vi "trace_init.vi"() -> (1 "Init seq.":string)   [LabVIEW 2021]
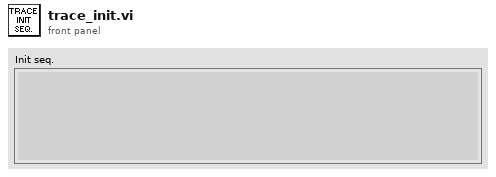
[diagram p1: front panel]
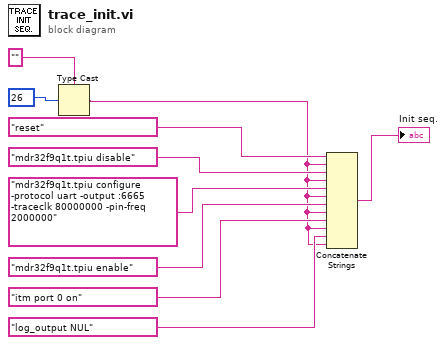
[diagram p0: block diagram]
diagram:
  n1 = Type Cast(type="", x=u8 26) -> (*(type *) &x=w1:string)
  n2 = Concatenate Strings("reset" ("data in"), w1, "mdr32f9q1t.tpiu disable" ("data in"), w1, "mdr32f9q1t.tpiu configure -protocol uart -output :6665 -traceclk 80000000 -pin-freq 2000000" ("data in"), w1, "mdr32f9q1t.tpiu enable" ("data in"), w1, "itm port 0 on" ("data in"), w1, "log_output NUL" ("data in"), w1) -> (→"Init seq.":string)
